vi "Vision Processing.vi"   [LabVIEW 2015]
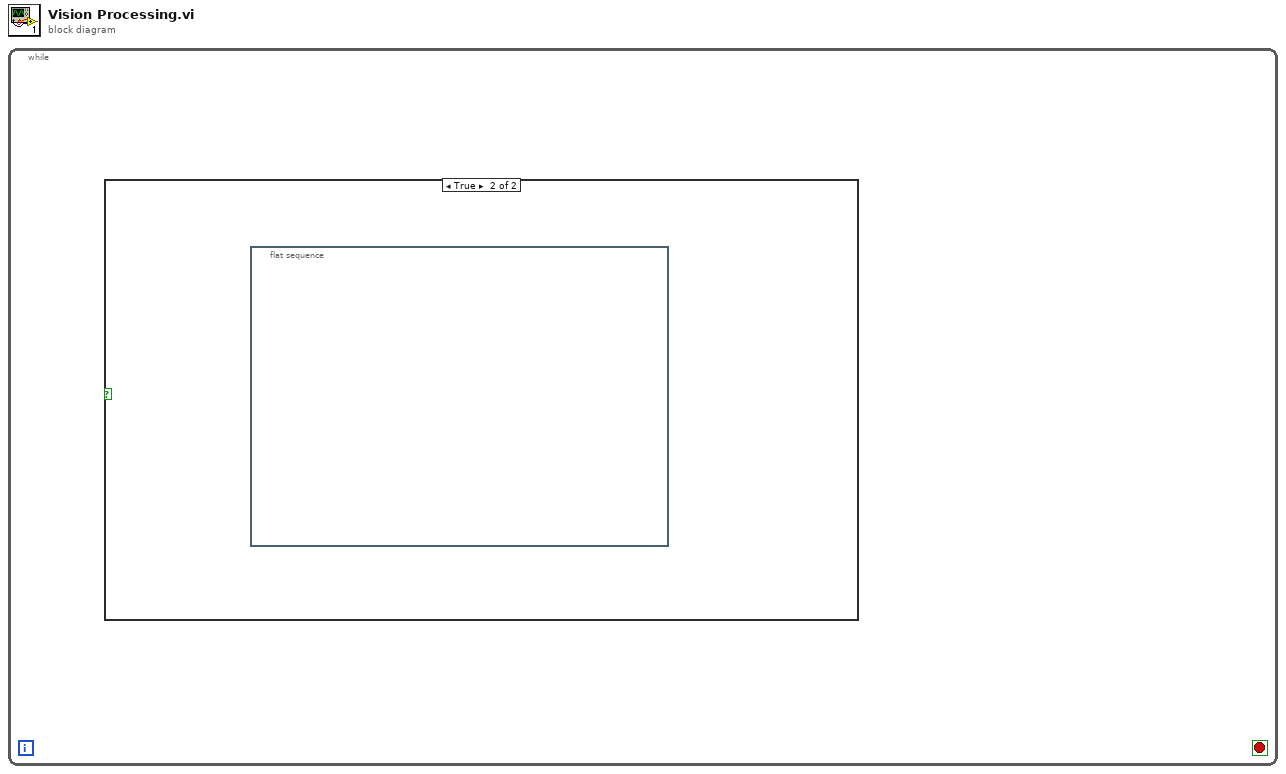
[diagram p0: block diagram]
diagram:
  n1 = while {
    stop <- _ stop-if-true
    n2 = case shown="True" {
      selector: _ -> [_ _]
      frame False {
      }
      frame True {
        n3 = flat-sequence {
          frame #0 {
          }
        }
      }
    }
  }
